vi "GetPath.vi"(11 "RVCLibrary_Bug2 in":refnum<class "RVCLibrary_Bug2.lvclass">) -> (0 "path cost":dbl, 1 "valid path":bool, 2 "path":refnum<data-value>[](array[refnum]), 3 "RVCLibrary_Bug2 out":refnum<class "RVCLibrary_Bug2.lvclass">)   [LabVIEW 2013, in "RVCLibrary_Bug2.lvclass"]
uses:
  RVCLibrary_Bug2.lvclass
  <vilib>/robotics/Navigation/shared/MapNode/AbstractDstarNode/NI_Robotics_AbstractDstarNode.lvclass
  RVCLibrary_Bug2.lvclass/RVCLibrary_Bug2.ctl
  <vilib>/robotics/Navigation/shared/MapNode/AbstractMapNode/NI_Robotics_AbstractMapNode.lvclass
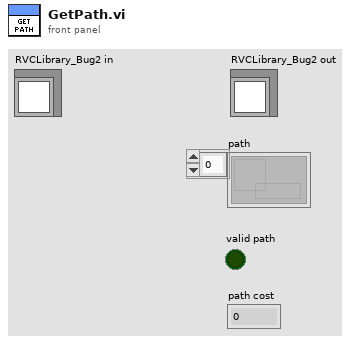
[diagram p1: front panel]
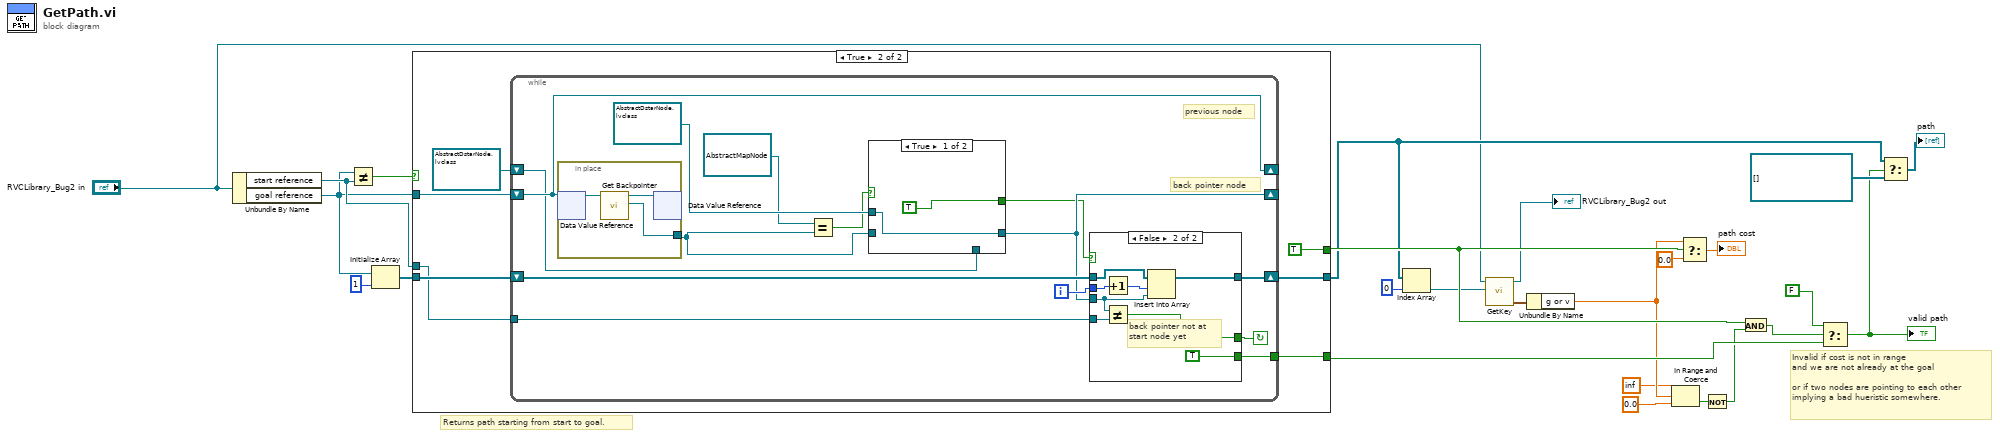
[diagram p0: block diagram]
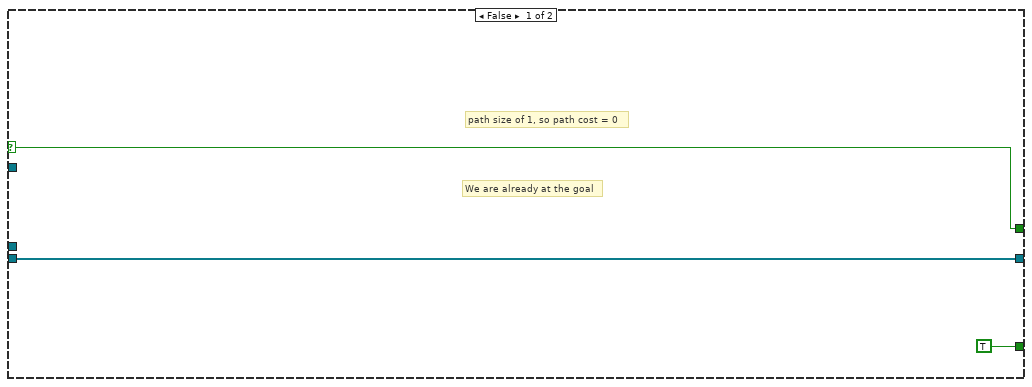
[diagram p2: hidden frame]
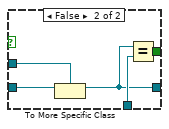
[diagram p3: hidden frame]
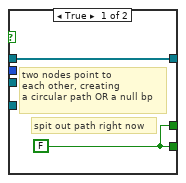
[diagram p4: hidden frame]
diagram:
  # "Invalid if cost is not in range\nand we are not already at the goal\n\nor if two nodes are pointing to each other\nimplying a bad hueristic somewhere."
  # "Returns path starting from start to goal."
  n1 = Unbundle By Name("RVCLibrary_Bug2 in") -> ("start reference"=w22:refnum<data-value>, "goal reference"=w21:refnum<data-value>)
  n2 = Not Equal?(x=w21, y=w22) -> (x != y?=w25:bool)
  n3 = Initialize Array(w21, 1 ("dimension size")) -> (w24:refnum<data-value>[])
  n4 = case shown="True" w25 {
    selector: w25 -> [w26 _]
    tunnel: w21 -> [_ w35]
    tunnel: w24 -> [w28 w34]
    tunnel: [w28 w33] -> w4
    tunnel: w22 -> [_ w32]
    tunnel: [TRUE ("valid path") w30] -> w19
    tunnel: [w26 TRUE] -> w14
    frame False {
      # "We are already at the goal"
      # "path size of 1, so path cost = 0"
    }
    frame True {
      n5 = while {
        shift-right: [w41] -> _
        shift-left: w35 -> [w45]
        shift-right: [w46] -> w33
        shift-left: w34 -> [w49]
        tunnel: w32 -> [w43]
        shift-right: [w45] -> _
        shift-left: refnum<data-value> refnum ("start node reference") -> [w37]
        tunnel: [w44] -> w30
        i -> [w48]
        stop <- w42 continue-if-true
        # "previous node"
        # "back pointer node"
        n6 = in-place {
          in-place-border: [w67] -> w39
          n7 = in-place-dvr #1(w45) -> (w69:refnum<class "NI_Robotics_AbstractDstarNode.lvclass">)  [unwired: 1 out]
          n8 = call <vilib>:"Get Backpointer.vi"("AbstractDstarNode in"=w69) -> ("BackPointer"=w67:refnum<data-value>, "AbstractDstarNode out"=w68:refnum<class "NI_Robotics_AbstractDstarNode.lvclass">)  [unwired: 8 in, 1 out]
          n9 = in-place-dvr #1(w68) -> ()  [unwired: 2 out]
        }
        n10 = Equal?(x=refnum<data-value> refnum ("BackPointer"), y=w39) -> (x = y?=w38:bool)
        n11 = case shown="True" w38 {
          tunnel: refnum<data-value> refnum ("goal node reference") -> [w51 w56]
          tunnel: [w51 w53] -> w41
          tunnel: w39 -> [_ w55]
          tunnel: w37 -> [_ w54]
          tunnel: [TRUE ("valid path") w52] -> w36
          frame True {
          }
          frame False {
            n12 = To More Specific Class(target class=w56, reference=w55) -> (specific class reference=w53:refnum<data-value>)  [unwired: 1 in, 1 out]
            n13 = Equal?(x=w53, y=w54) -> (x = y?=w52:bool)
          }
        }
        n14 = case shown="False" w36 {
          tunnel: w49 -> [w58 w66]
          tunnel: w48 -> [_ w65]
          tunnel: [w58 w63] -> w46
          tunnel: w41 -> [_ w61]
          tunnel: [w57 TRUE ("valid path")] -> w44
          tunnel: w43 -> [_ w60]
          tunnel: [w57 w59] -> w42
          frame True {
            w57 = FALSE ("valid path")
            # "two nodes point to\neach other, creating\na circular path OR a null bp"
            # "spit out path right now"
          }
          frame False {
            # "back pointer not at\nstart node yet"
            n15 = Increment(x=w65) -> (x+1=w64:i32)
            n16 = Not Equal?(x=w61, y=w60) -> (x != y?=w59:bool)
            n17 = Insert Into Array(array=w66, index=w64, new element=w61) -> (w63:refnum<data-value>[])
          }
        }
      }
    }
  }
  n18 = Index Array(array=w4, index=0) -> (element=w13:refnum<data-value>)
  n19 = call "GetKey.vi"("node ref in"=w13, "RVCLibrary_Bug2 in"="RVCLibrary_Bug2 in") -> ("key out"=w12:cluster{"(g or v) + h":dbl, "g or v":dbl}, "RVCLibrary_Bug2 out"=→"RVCLibrary_Bug2 out":refnum<class "RVCLibrary_Bug2.lvclass">)  [unwired: 7 in, 1 out]
  n20 = Unbundle By Name(w12) -> ("g or v"=w11:dbl)
  n21 = In Range and Coerce(upper limit=inf, x=w11, lower limit=0.0) -> (In Range?=w8:bool)  [unwired: 1 out]
  n22 = Select(t=w11, s=w14, f=0.0) -> (s? t:f=→"path cost":dbl)
  n23 = Not(x=w8) -> (.not. x?=w7:bool)
  n24 = And(x=w14, y=w7) -> (x .and. y?=w15:bool)
  n25 = Select(t=FALSE, s=w15, f=w19) -> (s? t:f=w5:bool)
  "valid path" <- w5
  n26 = Select(t=w4, s=w5, f=refnum<data-value>[] []) -> (s? t:f=→"path":refnum<data-value>[])
